vi "Line Configuration Dialog.vi"(8 "error in":errorcluster, 9 "engine configuration in":refnum<class "engine configuration.lvclass">, 10 "tag bus configurable plugin module configuration":refnum<class "SystemLink File configuration.lvclass">, 11 "Line":T4) -> (0 "error out":errorcluster, 1 "success":bool, 2 "changed":bool, 3 "Mappings out":T3)   [LabVIEW 2015, in "SystemLink File editor node.lvclass"]
doc: "A dialog for allowing a user to specify the values of a new line."
uses:
  SystemLink File editor node.lvclass
  module/configuration/Line.ctl
  <vilib>/NI/Tag Bus Module Framework/channel/TBM channel.lvclass
  module/configuration/Data Tag Type.ctl
  Mappings.ctl
  Map.ctl
  module/configuration/permissions.ctl
  <vilib>/NI/Module Execution Interface/Engine Configuration/engine configuration.lvclass
  module/configuration/SystemLink File configuration.lvclass
  <vilib>/NI/Tag Bus Module Framework/channel/TBM channel.lvclass/TBM channel.ctl
  <vilib>/NI/Tag Bus/tag/tag descriptor.lvclass/tag descriptor.ctl
  <vilib>/NI/Configuration Framework/serializable configuration/NISE_CEF_serializable configuration.lvclass/NISE_CEF_serializable configuration.ctl
  <vilib>/NI/Tag Bus/tag/write tag name.vi
  <vilib>/NI/Tag Bus Module Framework/channel/Write channel classification.vi
  <vilib>/NI/Tag Bus/tag/write data type.vi
  <vilib>/NI/Configuration Framework/serializable configuration/Read UID.vi
  <vilib>/NI/Tag Bus Module Framework/channel/Read channel classification.vi
  <vilib>/NI/Tag Bus/tag/read data type.vi
  <vilib>/Utility/LVClass/Get LV Class Name.vi
  <vilib>/NI/Configuration Framework/error generator/NISE_error generator.vi
  <vilib>/NI/Tag Bus/tag/tag descriptor.lvclass
  <vilib>/NI/DCAF UI Toolkit/Controls/DCAF UI Elements.lvlib
panel:
  in  "Data Tag Type":T1
  out "errors":string
  in  "Access Type":T2
  in  "Tag":i32(listbox)
  in  "Data Type":i32(listbox)
  in  "Systemlink Tag":string
  in  "cancel":bool
  in  "ok":bool
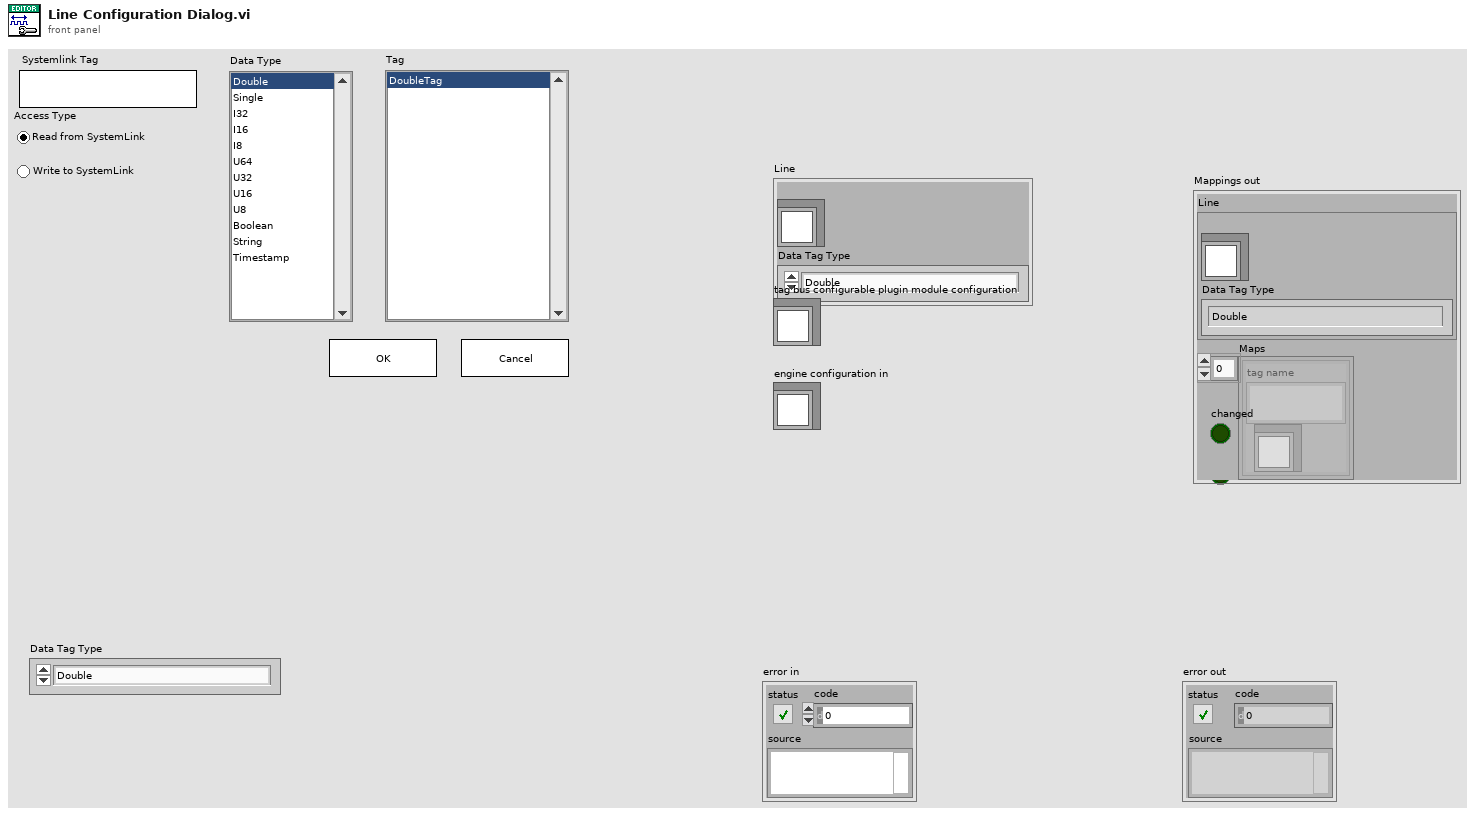
[diagram p1: front panel]
types:
  T1 = typedef "SystemLink File configuration.lvclass/Data Tag Type.ctl" = enum16{"Double", "Single", "I32", "I16", "I8", "U64", "U32", "U16", "U8", "Boolean", "String", "Timestamp"}
  T2 = typedef "SystemLink File configuration.lvclass/permissions.ctl" = enum32{"Read from SystemLink", "Write to SystemLink"}
  T3 = typedef "SystemLink File editor node.lvclass/Mappings.ctl" = cluster{"Line":T4, "Maps":T5[]}
  T4 = typedef "SystemLink File configuration.lvclass/Line.ctl" = cluster{"channel":refnum<class "TBM channel.lvclass">, "Data Tag Type":T1}
  T5 = typedef "SystemLink File editor node.lvclass/Map.ctl" = cluster{"channel":refnum<class "TBM channel.lvclass">, "tag name":string}
  T6 = typedef "tag bus.lvlib/tag descriptor.lvclass/Data Type.ctl" = enum16{"Double", "Single", "I64", "I32", "I16", "I8", "U64", "U32", "U16", "U8", "Boolean", "String", "Array of Double", "Array of Single", "Array of I64", "Array of I32", "Array of I16", "Array of I8", "Array of U64", "Array of U32", "Array of U16", "Array of U8", "Array of Boolean", "Array of String"}
  T7 = typedef "TBM channel.lvclass/channel classification.ctl" = enum16{"input data", "output data", "processing parameter", "processing result"}
  T8 = enum8{"Enabled", "Disabled", "Disabled and Grayed Out"}
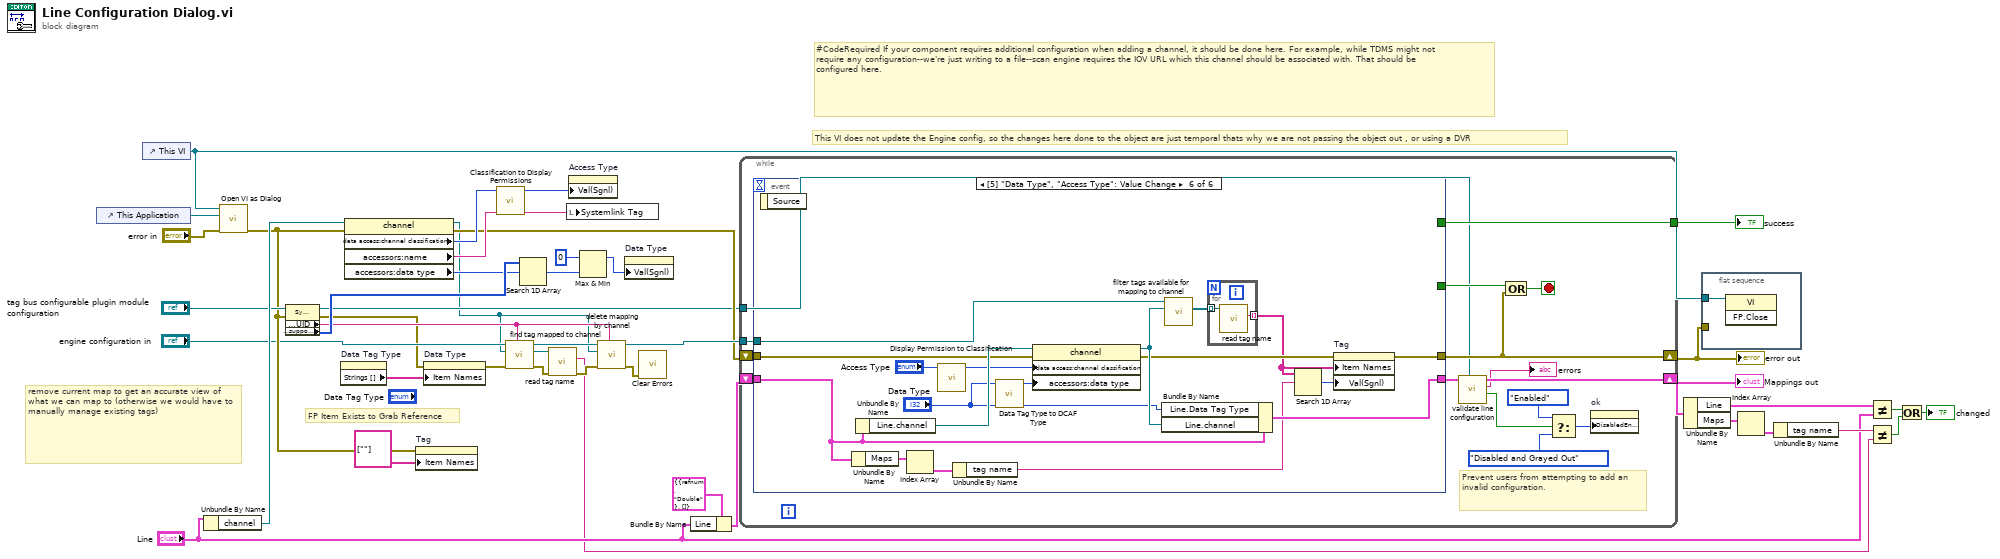
[diagram p0: block diagram]
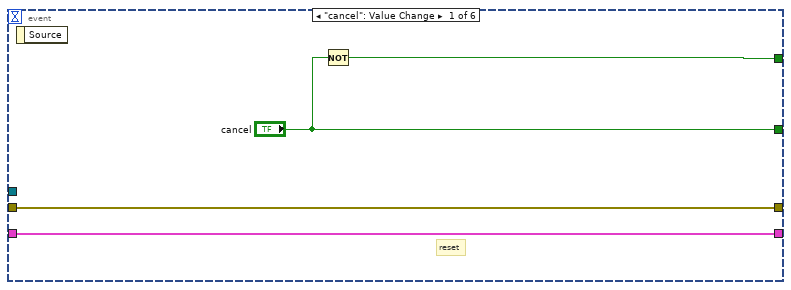
[diagram p2: hidden frame]
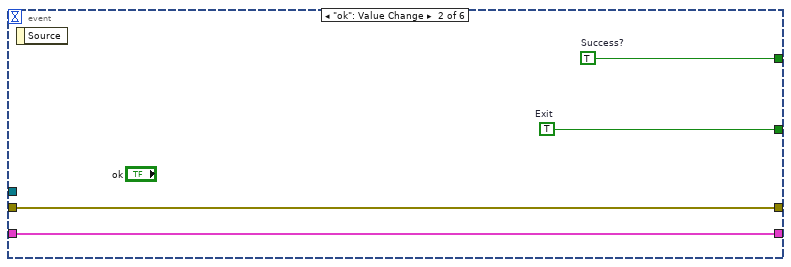
[diagram p3: hidden frame]
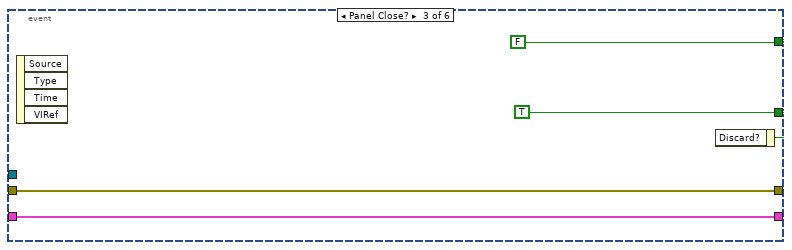
[diagram p4: hidden frame]
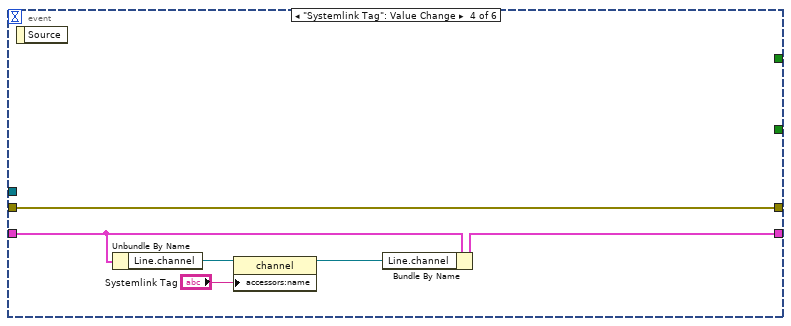
[diagram p5: hidden frame]
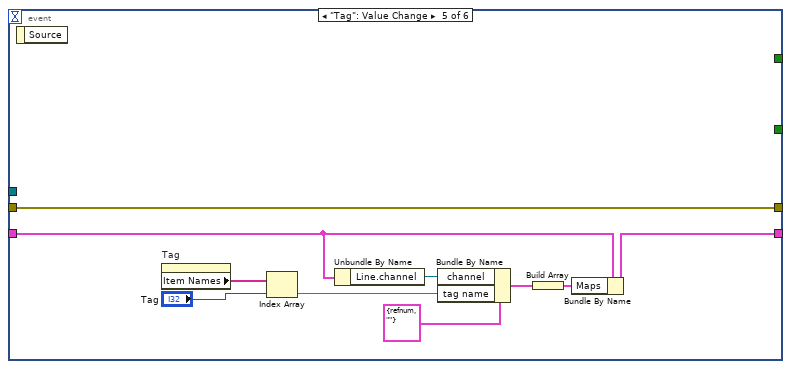
[diagram p6: hidden frame]
diagram:
  # "FP Item Exists to Grab Reference"
  # "This VI does not update the Engine config, so the changes here done to the object are just temporal thats why we are not passing the object out , or using a DVR"
  # "remove current map to get an accurate view of what we can map to (otherwise we would have to manually manage existing tags)"
  # "#CodeRequired If your component requires additional configuration when adding a channel, it should be done here. For example, while TDMS might not require any configuration--we're just writing to a file--scan engine requires the IOV URL which this channel should be associated with. That should be configured here."
  n1 = control-ref of="This Application"() -> (w27:refnum<vi>)
  n2 = control-ref of="This VI"() -> (w4:refnum<vi>)
  n3 = Unbundle By Name("Line") -> ("channel"=w37:refnum<class "TBM channel.lvclass">)
  n4 = call <vilib>:"Open VI as Dialog.vi"("error in (no error)"="error in", "This Application"=w27, "VI in"=w4) -> ("error out"=w25:errorcluster)  [unwired: 8 in]
  n5 = property class="SystemLin Tag Module configurat"(reference="tag bus configurable plugin module configuration", error in=w25) -> (reference out=w19:refnum<class "SystemLink File configuration.lvclass">, error out=w21:errorcluster, "Properties:UID"=w24:string, "Customize:Properties:supported types"=w41:T6[])
  n6 = property on="Data Tag Type" class="Enum (strict)"() -> ("Strings []"=w1:string[])  [unwired: 2 in, 2 out]
  n7 = property class="channel"(reference=w37, error in=w25) -> (reference out=w17:refnum<class "TBM channel.lvclass">, error out=w20:errorcluster, "data access:channel classification"=w39:T7, "accessors:name"=w38:string, "accessors:data type"=w34:T6)
  n8 = property on="Tag" class="LstBox (strict)"(error in=w25, "Item Names"=string[] [""]) -> ()  [unwired: 1 in, 2 out]
  n9 = property on="Data Type" class="LstBox (strict)"(error in=w21, "Item Names"=w1) -> (error out=w18:errorcluster)  [unwired: 1 in, 1 out]
  n10 = call "Classification to Display Permissions.vi"("channel classification"=w39) -> ("permissions"=w35:T2)  [unwired: 10 in]
  n11 = call <vilib>:"find tag mapped to channel.vi"("owner"=w24, "error in"=w18, "channel"=w17, "engine configuration in"="engine configuration in") -> ("error out"=w12:errorcluster, "tag"=w13:refnum<class "tag descriptor.lvclass">, "engine configuration out"=w22:refnum<class "engine configuration.lvclass">)  [unwired: 5 in]
  n12 = Search 1D Array(1D array=w41, element=w34) -> (index of element=w16:i32)  [unwired: 1 in]
  n13 = call <vilib>:"read tag name.vi"("error in"=w12, "system tag in"=w13) -> ("error out"=w11:errorcluster, "name"=w2:string)  [unwired: 7 in, 1 out]
  n14 = local write "Systemlink Tag"(w38) -> ()
  n15 = property on="Access Type" class="RadioBtnsControl (strict)"("Val(Sgnl)"=w35) -> ()  [unwired: 2 in, 2 out]
  n16 = Max & Min(x=0 ("f"), y=w16) -> (max(x,y)=w14:i32)  [unwired: 1 out]
  n17 = call <vilib>:"delete mapping by channel.vi"("owner ID"=w24, "error in"=w11, "channel"=w17, "engine configuration in"=w22) -> ("error out"=w33:errorcluster, "engine configuration out"=w42:refnum<class "engine configuration.lvclass">)  [unwired: 6 in]
  n18 = property on="Data Type" class="LstBox (strict)"("Val(Sgnl)"=w14) -> ()  [unwired: 2 in, 2 out]
  n19 = call <vilib>:"Clear Errors.vi"("error in (no error)"=w33) -> ()  [unwired: 5 in, 2 out]
  n20 = Bundle By Name(cluster=T3 {"Line"={"channel"=refnum, "Data Tag Type"=enum."Double"}, "Maps"=[]} ("Mappings out"), "Line"="Line") -> (w30:T3)
  n21 = while {
    shift-right: [w50] -> w40
    shift-left: w20 -> [w57]
    tunnel: [w56] -> w43
    shift-right: [w51] -> w28
    shift-left: w30 -> [w53]
    tunnel: w42 -> [w58]
    tunnel: w19 -> [w45]
    stop <- w54 stop-if-true
    # "Prevent users from attempting to add an invalid configuration."
    n22 = event shown="[5] \"Data Type\", \"Access Type\": Value Change" {
      selector: _ -> [_ _ _ _ _ _]
      dyn-events: _ -> [_ _ _ _ _ _]
      timeout: _ -> [_ _ _ _ _ _]
      tunnel: w58 -> [_ _ _ _ _ w91]
      tunnel: w57 -> [w62 w66 w70 w76 w86 w99]
      tunnel: [w62 w66 w70 w76 w86 w97] -> w50
      tunnel: [w61 w63 FALSE _ _ _] -> w56
      tunnel: ["cancel" w64 w68 _ _ _] -> w55
      tunnel: w53 -> [w59 w65 w67 w74 w81 w90]
      tunnel: [w59 w65 w67 w75 w78 w102] -> w52
      event "cancel": Value Change {
        # "reset"
        n23 = event-data() -> ()  [unwired: 1 in, 1 out]
        n24 = Not(x="cancel") -> (.not. x?=w61:bool)
      }
      event "ok": Value Change {
        w63 = TRUE  # Success?
        w64 = TRUE  # Exit
        n25 = event-data() -> ()  [unwired: 1 in, 1 out]
      }
      event Panel Close? {
        w68 = TRUE ("cancel")
        n26 = event-data() -> ()  [unwired: 1 in, 4 out]
        n27 = event-data("Discard?"=w68) -> ()  [unwired: 1 in, 1 out]
      }
      event "Systemlink Tag": Value Change {
        n28 = event-data() -> ()  [unwired: 1 in, 1 out]
        n29 = Unbundle By Name(w74) -> ("Line.channel"=w73:refnum<class "TBM channel.lvclass">)
        n30 = property class="channel"(reference=w73, "accessors:name"="Systemlink Tag") -> (reference out=w72:refnum<class "TBM channel.lvclass">)  [unwired: 1 in, 1 out]
        n31 = Bundle By Name(cluster=w74, "Line.channel"=w72) -> (w75:T3)
      }
      event "Tag": Value Change {
        n32 = event-data() -> ()  [unwired: 1 in, 1 out]
        n33 = property on="Tag" class="LstBox (strict)"() -> ("Item Names"=w84:string[])  [unwired: 2 in, 2 out]
        n34 = Index Array(array=w84, index="Tag") -> (element=w77:string)
        n35 = Unbundle By Name(w81) -> ("Line.channel"=w82:refnum<class "TBM channel.lvclass">)
        n36 = Bundle By Name(cluster=T5 {"channel"=refnum, "tag name"=""} ("Map"), "channel"=w82, "tag name"=w77) -> (w80:T5)
        n37 = Build Array(w80) -> (w79:T5[])
        n38 = Bundle By Name(cluster=w81, "Maps"=w79) -> (w78:T3)
      }
      event "Data Type": Value Change {
        n39 = event-data() -> ()  [unwired: 1 in, 1 out]
        n40 = Unbundle By Name(w90) -> ("Maps"=w94:T5[])
        n41 = Unbundle By Name(w90) -> ("Line.channel"=w104:refnum<class "TBM channel.lvclass">)
        n42 = Index Array(array=w94) -> (element=w93:T5)  [unwired: 1 in]
        n43 = call "Display Permission to Classification.vi"("display permissions"="Access Type") -> ("channel classification"=w89:T7)  [unwired: 10 in]
        n44 = Unbundle By Name(w93) -> ("tag name"=w92:string)
        n45 = call "Data Tag Type to DCAF Type.vi"("Data Tag Type"="Data Type") -> ("DCAF Data Type"=w88:T6)  [unwired: 10 in]
        n46 = property class="channel"(reference=w104, error in=w99, "data access:channel classification"=w89, "accessors:data type"=w88) -> (reference out=w103:refnum<class "TBM channel.lvclass">, error out=w98:errorcluster)
        n47 = Bundle By Name(cluster=w90, "Line.Data Tag Type"="Data Type", "Line.channel"=w103) -> (w102:T3)
        n48 = call-dynamic "filter tags available for mapping to channel.vi"("channel to map to"=w103, "engine configuration in"=w91) -> ("filtered tags"=w101:refnum<class "tag descriptor.lvclass">[])  [unwired: 8 in, 1 out]
        n49 = for {
          tunnel: w101 -> [w106] mode=indexing
          tunnel: [w105] -> w96 mode=indexing
          n50 = call <vilib>:"read tag name.vi"("system tag in"=w106) -> ("name"=w105:string)  [unwired: 8 in, 2 out]
        }
        n51 = Search 1D Array(1D array=w96, element=w92) -> (index of element=w95:i32)  [unwired: 1 in]
        n52 = property on="Tag" class="LstBox (strict)"(error in=w98, "Item Names"=w96, "Val(Sgnl)"=w95) -> (error out=w97:errorcluster)  [unwired: 1 in, 1 out]
      }
    }
    n53 = call "validate line configuration.vi"("Module Config"=w45, "Mappings in"=w52) -> ("valid?"=w49:bool, "errors"=→"errors":string, "Mappings out"=w51:T3)  [unwired: 7 in]
    n54 = Compound Arithmetic op=OR(w55, w50) -> (w54:bool)
    n55 = Select(t=T8."Enabled" ("Disabled"), s=w49, f=T8."Disabled and Grayed Out") -> (s? t:f=w46:T8)
    n56 = property on="ok" class="Bool"("DisabledEnum"=w46) -> ()  [unwired: 2 in, 2 out]
  }
  "error out" <- w40
  "success" <- w43
  "Mappings out" <- w28
  n57 = Unbundle By Name(w28) -> ("Line"=w29:T4, "Maps"=w10:T5[])
  n58 = flat-sequence {
    tunnel: w40 -> [_]
    tunnel: w4 -> [w107]
    frame #0 {
      n59 = invoke class="VI" method="FP.Close"(reference=w107) -> ()  [unwired: 2 in, 3 out]
    }
  }
  n60 = Index Array(array=w10) -> (element=w9:T5)  [unwired: 1 in]
  n61 = Unbundle By Name(w9) -> ("tag name"=w8:string)
  n62 = Not Equal?(x=w29, y="Line") -> (x != y?=w6:bool)
  n63 = Not Equal?(x=w8, y=w2) -> (x != y?=w7:bool)
  n64 = Or(x=w6, y=w7) -> (x .or. y?=→"changed":bool)
